vi "Database Fetching.vi"() -> ()   [LabVIEW 2018]
doc: "This example fetches data from the specified table in a database named LabVIEW.mdb located in the LabVIEW examples>>database directory.\n\nThe table is assumed to be in the same format with the same datatypes as defined by the fetchdata table. You can use the Next and Previous buttons to move from the current record in the database table to the next or previous record."
uses:
  database example subvis/Fetching - State.ctl
  <vilib>/addons/database/Recordset.llb/Rec ObjectReference.ctl
  <vilib>/addons/database/Auxilliary.llb/DB Tools Cursor Type.ctl
  <vilib>/addons/database/Connection.llb/DB Tools Open Connec (Path).vi
  <vilib>/addons/database/Connection.llb/Conn Execute.vi
  <vilib>/addons/database/Recordset.llb/Rec Get Recordset Properties (R).vi
  <vilib>/addons/database/Recordset.llb/Rec Move To Next Record (R).vi
  <vilib>/addons/database/Recordset.llb/Rec Move To Previous Record (R).vi
  <vilib>/addons/database/Recordset.llb/Rec Fetch Integer Data (R).vi
  <vilib>/addons/database/Recordset.llb/Rec Fetch String Data (R).vi
  <vilib>/addons/database/Recordset.llb/Rec Fetch Binary Data (R).vi
  <vilib>/addons/database/Recordset.llb/Rec Destroy - Connection.vi
  <vilib>/addons/database/_DB Variant To Data/Database Variant To Data.xnode
  <vilib>/addons/database/NI_Database_API.lvlib
panel:
  in  "table":string(combo)="fetchdata"
  out "record number":i32
  in  "Stop":bool
  out "Phone Number":string
  out "Customer Number":i32
  out "Last Name":string
  out "First Name":string
  in  "Previous Record":bool
  in  "Next Record":bool
  # "Overview: Demonstrates how to fetch data from a database.\nRequirements: Database Connectivity Toolkit\nInstructions:\n1. Run the VI.\n2. Click the Previous Record and Next Record buttons to fetch individual records from the database.\n3. Click Stop to stop the VI.\n4. Specify the 'fetchempty' value for the table and run the VI again to see how an empty table is detected."
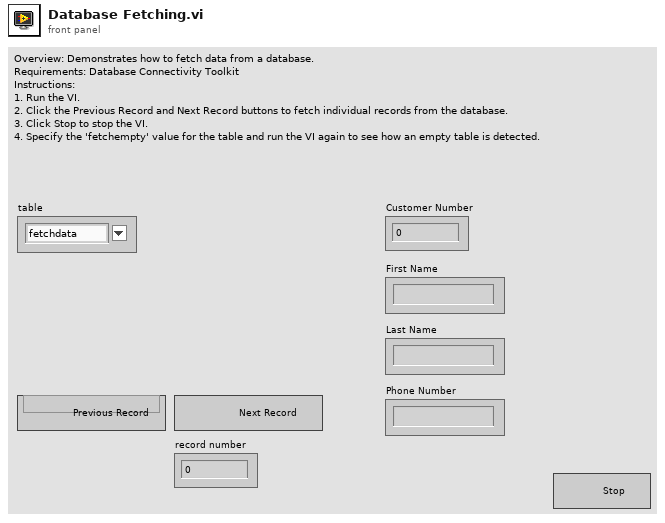
[diagram p1: front panel]
types:
  T1 = typedef "NI_Database_API.lvlib/Rec ObjectReference.ctl" = refnum<k1>
  T2 = typedef "Fetching - State.ctl" = enum16{"Initialize", "Wait for Event", "Prepare for Next", "Prepare for Previous", "Query Database", "Exit"}
  T3 = typedef "NI_Database_API.lvlib/DB Tools Cursor Type.ctl" = enum16{"forward-only", "keyset", "dynamic", "static"}
  T4 = typedef "NI_Database_API.lvlib/Conn ObjectReference.ctl" = refnum<k1>
  T5 = typedef "NI_Database_API.lvlib/Rec Properties.ctl" = cluster{"column count":i32, "record index":i32, "record count":i32, "bof?":bool, "eof?":bool, "cursor type":T3, "cache size":i32, "state":enum16{"closed", "open"}}
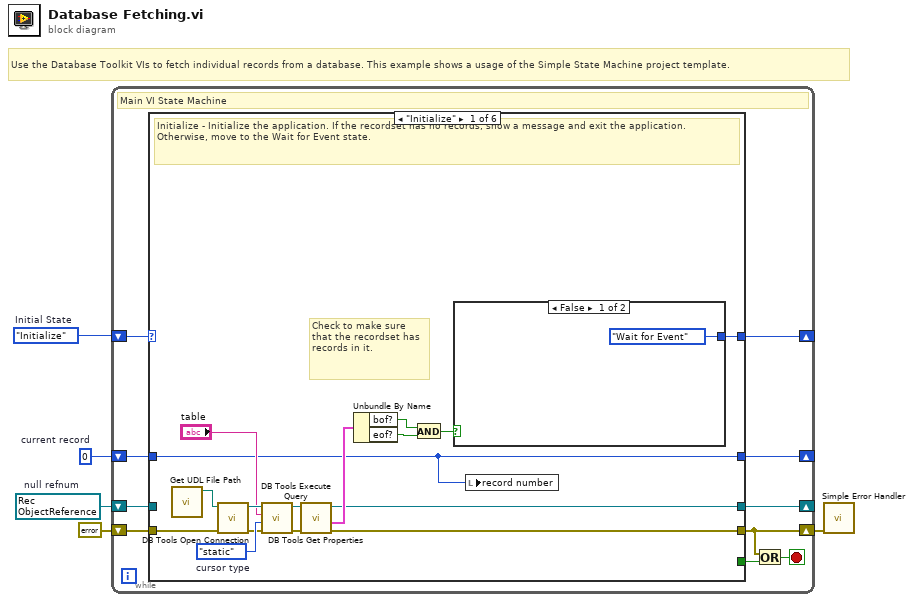
[diagram p0: block diagram]
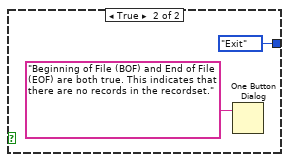
[diagram p2: hidden frame]
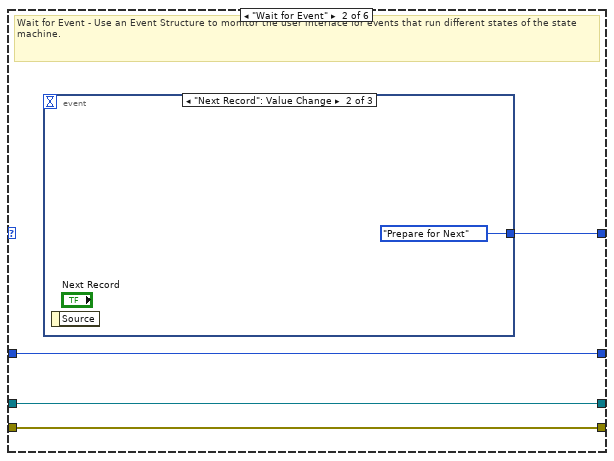
[diagram p3: hidden frame]
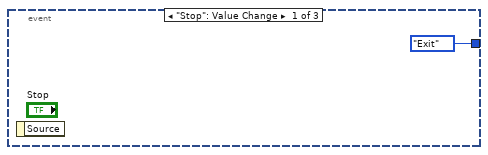
[diagram p4: hidden frame]
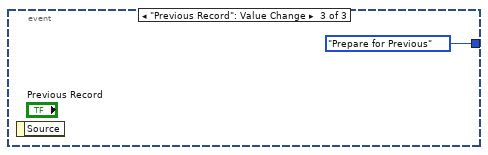
[diagram p5: hidden frame]
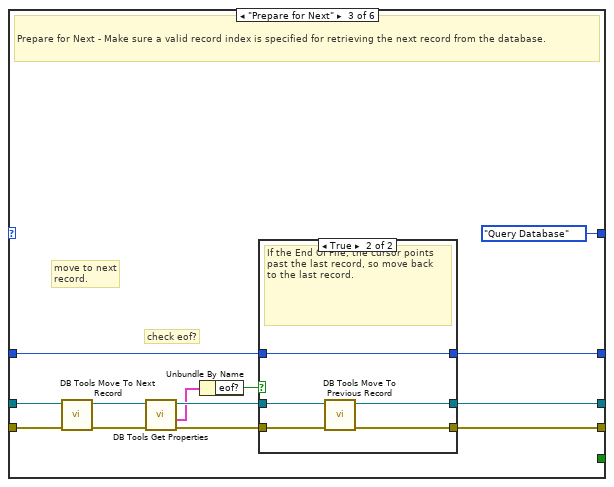
[diagram p6: hidden frame]
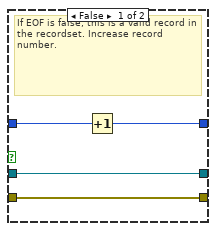
[diagram p7: hidden frame]
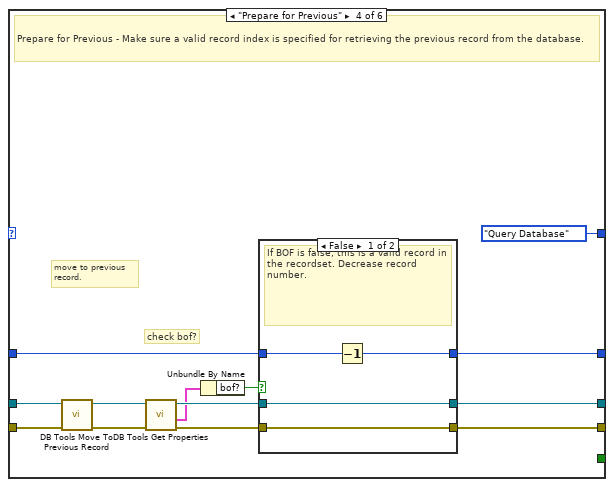
[diagram p8: hidden frame]
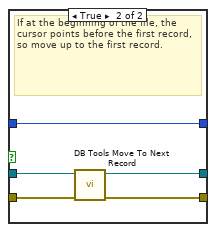
[diagram p9: hidden frame]
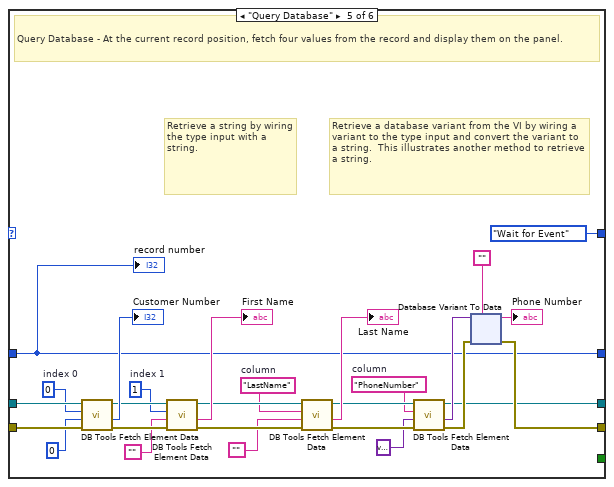
[diagram p10: hidden frame]
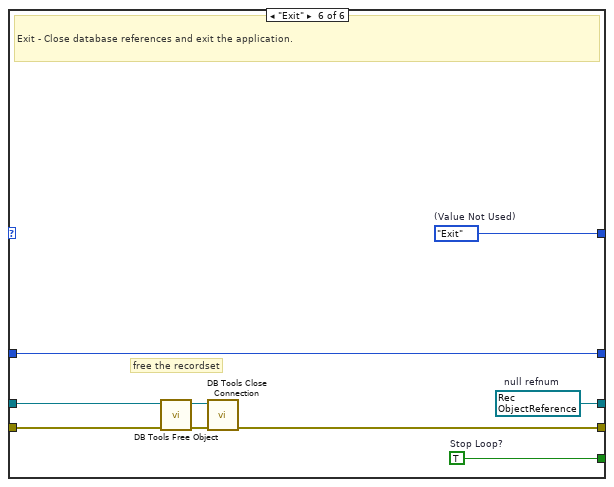
[diagram p11: hidden frame]
diagram:
  w1 = 0  # current record
  w2 = T1 refnum items=["Recordset"]  # null refnum
  w3 = Fetching_-_State."Initialize"  # Initial State
  # "Use the Database Toolkit VIs to fetch individual records from a database. This example shows a usage of the Simple State Machine project template."
  n1 = while {
    shift-right: [w14] -> _
    shift-left: w3 -> [w15]
    shift-right: [w10] -> w5
    shift-left: errorcluster {"status"=FALSE, "code"=0, "source"=""} ("error constant") -> [w13]
    shift-right: [w9] -> _
    shift-left: w2 -> [w8]
    shift-right: [w6] -> _
    shift-left: w1 -> [w7]
    stop <- w11 stop-if-true
    # "Main VI State Machine"
    n2 = case shown="\"Initialize\"" w15 {
      tunnel: [w18 w38 Fetching_-_State."Query Database" ("(Value Not Used)") Fetching_-_State."Query Database" ("(Value Not Used)") Fetching_-_State."Wait for Event" ("(Value Not Used)") w153] -> w14
      tunnel: [_ _ _ _ _ w152] -> w12
      tunnel: w13 -> [w22 w36 w48 w70 w99 w149]
      tunnel: [w21 w36 w47 w69 w98 w148] -> w10
      tunnel: [w20 w37 w42 w64 w95 w146] -> w9
      tunnel: w8 -> [_ w37 w43 w65 w96 w147]
      tunnel: w7 -> [w16 w35 w46 w68 w97 w145]
      tunnel: [w16 w35 w44 w66 w97 w145] -> w6
      frame "Initialize" {
        w26 = DB_Tools_Cursor_Type."static"  # cursor type
        # "Check to make sure that the recordset has\nrecords in it."
        # "Initialize - Initialize the application. If the recordset has no records, show a message and exit the application. Otherwise, move to the Wait for Event state."
        n3 = call "Get UDL File Path.vi"() -> ("UDL file path"=w23:path)  [unwired: 11 in]
        n4 = call-poly <vilib>:"DB Tools Open Connection.vi"("error in (no error)"=w22, "connection information"=w23) -> ("error out"=w24:errorcluster, "connection reference"=w25:T4)  [unwired: 6 in]
        n5 = call-poly <vilib>:"DB Tools Execute Query.vi"("error in (no error)"=w24, "cursor type"=w26, "SQL query"="table", "connection reference"=w25) -> ("error out"=w28:errorcluster, "recordset reference"=w27:T1)  [unwired: 4 in]
        n6 = call-poly <vilib>:"DB Tools Get Properties.vi"("error in (no error)"=w28, "recordset reference"=w27) -> ("error out"=w21:errorcluster, "recordset properties"=w29:T5, "recordset reference out"=w20:T1)  [unwired: 3 in]
        n7 = Unbundle By Name(w29) -> ("bof?"=w31:bool, "eof?"=w30:bool)
        n8 = And(x=w31, y=w30) -> (x .and. y?=w19:bool)
        n9 = case shown="False" w19 {
          tunnel: [Fetching_-_State."Wait for Event" ("(Value Not Used)") Fetching_-_State."Exit" ("(Value Not Used)")] -> w18
          frame False {
          }
          frame True {
            n10 = One Button Dialog(message="Beginning of File (BOF) and End of File (EOF) are both true. This indicates that there are no records in the recordset.") -> ()  [unwired: 1 in, 1 out]
          }
        }
        n11 = local write "record number"(w16) -> ()
      }
      frame "Wait for Event" {
        # "Wait for Event - Use an Event Structure to monitor the user interface for events that run different states of the state machine."
        n12 = event shown="[1] \"Next Record\": Value Change" {
          selector: _ -> [_ _ _]
          dyn-events: _ -> [_ _ _]
          timeout: _ -> [_ _ _]
          tunnel: [Fetching_-_State."Exit" ("Next State") Fetching_-_State."Prepare for Next" ("Next State") Fetching_-_State."Prepare for Previous" ("Next State")] -> w38
          event "Stop": Value Change {
            n13 = event-data() -> ()  [unwired: 1 in, 1 out]
          }
          event "Next Record": Value Change {
            n14 = event-data() -> ()  [unwired: 1 in, 1 out]
          }
          event "Previous Record": Value Change {
            n15 = event-data() -> ()  [unwired: 1 in, 1 out]
          }
        }
      }
      frame "Prepare for Next" {
        # "check eof?"
        # "move to next\nrecord."
        # "Prepare for Next - Make sure a valid record index is specified for retrieving the next record from the database."
        n16 = call-poly <vilib>:"DB Tools Move To Next Record.vi"("error in (no error)"=w48, "recordset reference"=w43) -> ("error out"=w53:errorcluster, "recordset reference out"=w54:T1)  [unwired: 8 in]
        n17 = call-poly <vilib>:"DB Tools Get Properties.vi"("error in (no error)"=w53, "recordset reference"=w54) -> ("error out"=w52:errorcluster, "recordset properties"=w49:T5, "recordset reference out"=w51:T1)  [unwired: 3 in]
        n18 = Unbundle By Name(w49) -> ("eof?"=w50:bool)
        n19 = case shown="True" w50 {
          tunnel: w51 -> [w55 w63]
          tunnel: w52 -> [w56 w62]
          tunnel: w46 -> [w58 w61]
          tunnel: [w57 w61] -> w44
          tunnel: [w56 w60] -> w47
          tunnel: [w55 w59] -> w42
          frame False {
            # "If EOF is false, this is a valid record in the recordset. Increase record number."
            n20 = Increment(x=w58) -> (x+1=w57:i32)
          }
          frame True {
            # "If the End Of File, the cursor points\npast the last record, so move back \nto the last record."
            n21 = call-poly <vilib>:"DB Tools Move To Previous Record.vi"("error in (no error)"=w62, "recordset reference"=w63) -> ("error out"=w60:errorcluster, "recordset reference out"=w59:T1)  [unwired: 8 in]
          }
        }
      }
      frame "Prepare for Previous" {
        # "check bof?"
        # "move to previous\nrecord."
        # "Prepare for Previous - Make sure a valid record index is specified for retrieving the previous record from the database."
        n22 = call-poly <vilib>:"DB Tools Move To Previous Record.vi"("error in (no error)"=w70, "recordset reference"=w65) -> ("error out"=w75:errorcluster, "recordset reference out"=w76:T1)  [unwired: 8 in]
        n23 = call-poly <vilib>:"DB Tools Get Properties.vi"("error in (no error)"=w75, "recordset reference"=w76) -> ("error out"=w74:errorcluster, "recordset properties"=w71:T5, "recordset reference out"=w73:T1)  [unwired: 3 in]
        n24 = Unbundle By Name(w71) -> ("bof?"=w72:bool)
        n25 = case shown="False" w72 {
          tunnel: w73 -> [w77 w85]
          tunnel: w74 -> [w78 w84]
          tunnel: w68 -> [w80 w83]
          tunnel: [w79 w83] -> w66
          tunnel: [w78 w82] -> w69
          tunnel: [w77 w81] -> w64
          frame False {
            # "If BOF is false, this is a valid record in the recordset. Decrease record number."
            n26 = Decrement(x=w80) -> (x-1=w79:i32)
          }
          frame True {
            # "If at the beginning of the file, the \ncursor points before the first record, so move up to the first record."
            n27 = call-poly <vilib>:"DB Tools Move To Next Record.vi"("error in (no error)"=w84, "recordset reference"=w85) -> ("error out"=w82:errorcluster, "recordset reference out"=w81:T1)  [unwired: 8 in]
          }
        }
      }
      frame "Query Database" {
        w86 = "LastName"  # column
        w87 = "PhoneNumber"  # column
        w92 = 1  # index 1
        w93 = 0  # index 0
        # "Retrieve a database variant from the VI by wiring a variant to the type input and convert the variant to a string.  This illustrates another method to retrieve a string."
        # "Retrieve a string by wiring the type input with a string."
        # "Query Database - At the current record position, fetch four values from the record and display them on the panel."
        n28 = call-poly <vilib>:"DB Tools Fetch Element Data.vi"("error in (no error)"=w99, "type"=0, "column index"=w93, "recordset reference"=w96) -> ("error out"=w100:errorcluster, "data"=→"Customer Number":i32, "recordset reference out"=w101:T1)  [unwired: 3 in]
        n29 = call-poly <vilib>:"DB Tools Fetch Element Data.vi"("error in (no error)"=w100, "type"="", "column index"=w92, "recordset reference"=w101) -> ("error out"=w102:errorcluster, "data"=→"First Name":string, "recordset reference out"=w103:T1)  [unwired: 3 in]
        n30 = call-poly <vilib>:"DB Tools Fetch Element Data.vi"("error in (no error)"=w102, "type"="", "column index"=w86, "recordset reference"=w103) -> ("error out"=w104:errorcluster, "data"=→"Last Name":string, "recordset reference out"=w105:T1)  [unwired: 3 in]
        n31 = call-poly <vilib>:"DB Tools Fetch Element Data.vi"("error in (no error)"=w104, "type"=variant, "column index"=w87, "recordset reference"=w105) -> ("error out"=w107:errorcluster, "data"=w106:variant, "recordset reference out"=w95:T1)  [unwired: 3 in]
        n32 = xnode "Database Variant To Data"("database variant"=w106, "error in (no error)"=w107, "type"="") -> ("data"=→"Phone Number":string, "error out"=w98:errorcluster)
        "record number" <- w97
      }
      frame "Exit" {
        w146 = T1 refnum items=["Recordset"]  # null refnum
        w152 = TRUE  # Stop Loop?
        w153 = Fetching_-_State."Exit"  # (Value Not Used)
        # "free the recordset"
        # "Exit - Close database references and exit the application."
        n33 = call-poly <vilib>:"DB Tools Free Object.vi"("error in (no error)"=w149, "recordset reference"=w147) -> ("error out"=w151:errorcluster, "connection reference"=w150:T4)  [unwired: 8 in]
        n34 = call <vilib>:"DB Tools Close Connection.vi"("error in (no error)"=w151, "connection reference"=w150) -> ("error out"=w148:errorcluster)  [unwired: 5 in]
      }
    }
    n35 = Or(x=w10, y=w12) -> (x .or. y?=w11:bool)
  }
  n36 = call <vilib>:"Simple Error Handler.vi"("error in (no error)"=w5) -> ()  [unwired: 4 in, 5 out]
